vi "get_total_number_of_pixels_per_cycle.vi"(8 "error in (no error)":errorcluster, 11 "TrajectoryMG100122AODFrameScan in":refnum<class "TrajectoryMG100122AODFrameScan.lvclass">) -> (0 "error out":errorcluster, 2 "total number of pixels per cycle":i32, 3 "TrajectoryMG100122AODFrameScan out":refnum<class "TrajectoryMG100122AODFrameScan.lvclass">)   [LabVIEW 2010, in "TrajectoryMG100122AODFrameScan.lvclass"]
uses:
  TrajectoryMG100122AODFrameScan.lvclass
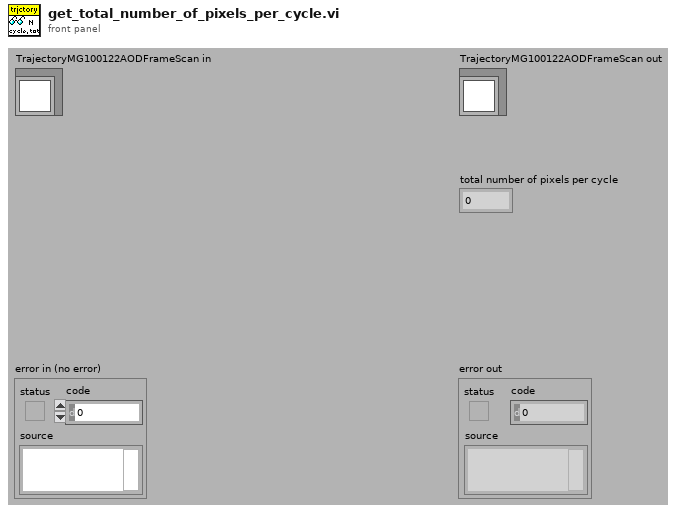
[diagram p1: front panel]
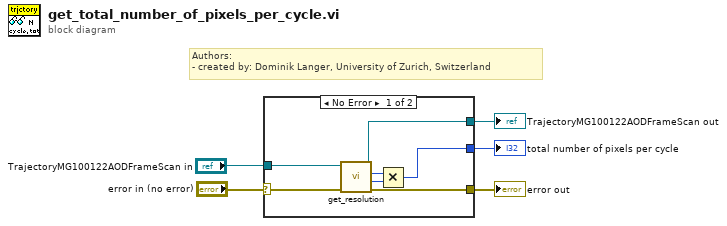
[diagram p0: block diagram]
diagram:
  # "Authors: \n- created by: Dominik Langer, University of Zurich, Switzerland"
  n1 = case shown="No Error" "error in (no error)" {
    selector: "error in (no error)" -> [w7 w13]
    tunnel: [w10 _] -> w5
    tunnel: "TrajectoryMG100122AODFrameScan in" -> [w9 w14]
    tunnel: [w8 w13] -> w3
    tunnel: [w6 w14] -> w1
    frame No Error {
      n2 = call-dynamic "get_resolution.vi"("error in (no error)"=w7, "TrajectoryMG100122AODFrameScan in"=w9) -> ("error out"=w8:errorcluster, "y resolution"=w11:i32, "x resolution"=w12:i32, "TrajectoryMG100122AODFrameScan out"=w6:refnum<class "TrajectoryMG100122AODFrameScan.lvclass">)  [unwired: 6 in]
      n3 = Multiply(x=w12, y=w11) -> (x*y=w10:i32)
    }
    frame Error {
    }
  }
  "error out" <- w3
  "TrajectoryMG100122AODFrameScan out" <- w1
  "total number of pixels per cycle" <- w5
